vi "Run Tests (Path).vi"(8 "error in (no error)":errorcluster, 10 "Project or Class Path":path, 11 "Execution API In":refnum<class "Execution API.lvclass">) -> (0 "error out":errorcluster, 3 "Execution API Out":refnum<class "Execution API.lvclass">)   [LabVIEW 2020, in "Execution API.lvclass"]
doc: "Run all tests in a project or a test case at the specified path."
uses:
  Execution API.lvclass
  LUnit Test Suite.lvclass
  <vilib>/Utility/error.llb/Error Cluster From Error Code.vi
  <vilib>/ErrorRing/Error Ring.xnode
  Execution API.lvclass/Execution API.ctl
  Framework/Test Finder/Test Finder.lvclass
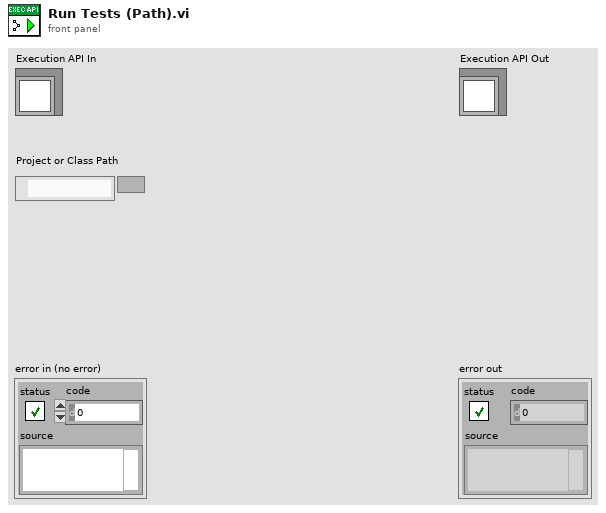
[diagram p1: front panel]
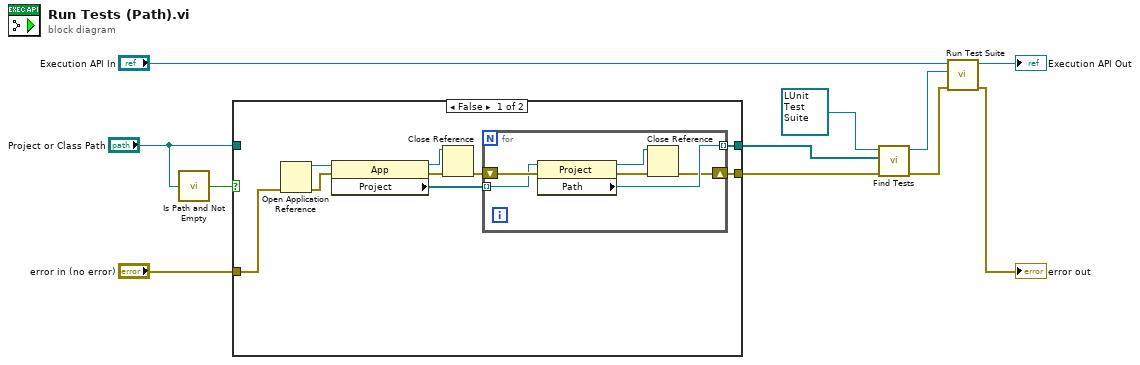
[diagram p0: block diagram]
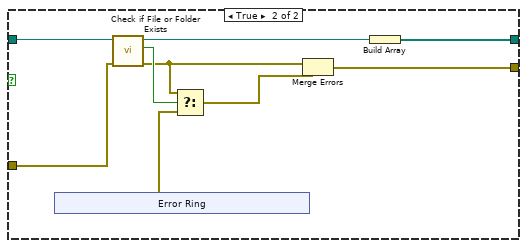
[diagram p2: hidden frame]
diagram:
  n1 = call <vilib>:"Is Path and Not Empty.vi"("path"="Project or Class Path") -> ("Is Path and Not Empty?"=w2:bool)  [unwired: 4 in]
  n2 = case shown="False" w2 {
    tunnel: "error in (no error)" -> [w18 w35]
    tunnel: [w16 w30] -> w6
    tunnel: "Project or Class Path" -> [_ w29]
    tunnel: [w14 w27] -> w1
    frame False {
      n3 = Open Application Reference(8:w18) -> (0:w17:errorcluster, 3:w20:refnum<vi>)  [unwired: 3 in]
      n4 = property class="App"(reference=w20, error in=w17) -> (reference out=w12:refnum<vi>, error out=w19:errorcluster, "Project"=w15:refnum<vi>[])
      n5 = Close Reference(reference=w12, error in (no error)=w19) -> (error out=w13:errorcluster)
      n6 = for {
        shift-right: [w22] -> w16
        shift-left: w13 -> [w26]
        tunnel: w15 -> [w24] mode=indexing
        tunnel: [w23] -> w14 mode=indexing
        n7 = property class="Project"(reference=w24, error in=w26) -> (reference out=w21:refnum<vi>, error out=w25:errorcluster, "Path"=w23:path)
        n8 = Close Reference(reference=w21, error in (no error)=w25) -> (error out=w22:errorcluster)
      }
    }
    frame True {
      n9 = xnode "Error Ring"() -> ("error out"=w31:errorcluster)
      n10 = call <vilib>:"Check if File or Folder Exists.vi"("error in (no error)"=w35, "path"=w29) -> ("error out"=w33:errorcluster, "file or folder exists?"=w34:bool, "dup path"=w28:path)  [unwired: 7 in]
      n11 = Select(t=w33, s=w34, f=w31) -> (s? t:f=w32:errorcluster)
      n12 = Merge Errors(w33, w32) -> (w30:errorcluster)
      n13 = Build Array(w28) -> (w27:path[])
    }
  }
  n14 = call "Find Tests.vi"("error in (no error)"=w6, "File Paths"=w1, "LUnit Test Suite"=refnum<class "LUnit Test Suite.lvclass"> refnum) -> ("error out"=w4:errorcluster, "LUnit Test Suite"=w5:refnum<class "LUnit Test Suite.lvclass">)  [unwired: 7 in]
  n15 = call "Run Test Suite.vi"("error in (no error)"=w4, "Test Suite"=w5, "Execution API In"="Execution API In") -> ("error out"=→"error out":errorcluster, "Execution API Out"=→"Execution API Out":refnum<class "Execution API.lvclass">)  [unwired: 7 in]
